vi "process_exit_callback.vi"(4 "ProcessExit event":refnum<user-event>, 5 "Event Data":cluster{"sender":refnum<k24>, "e":refnum<k24>}, 6 "Control Ref":refnum<k24>, 7 "Event Common Data":T1) -> ()   [LabVIEW 2019, in "dotnet_system_exec.lvclass"]
uses:
  dotnet_system_exec.lvclass
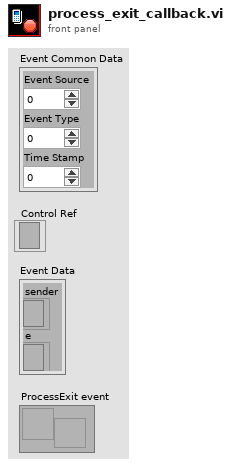
[diagram p1: front panel]
types:
  T1 = cluster{"Event Source":i32, "Event Type":u32, "Time Stamp":u32}
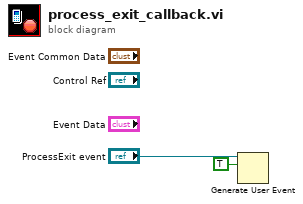
[diagram p0: block diagram]
diagram:
  n1 = Generate User Event(user event="ProcessExit event", event data cluster=TRUE ("event data")) -> ()  [unwired: 2 in, 2 out]
